vi "Decimate DFD (Array).vi"(8 "error in (no error)":errorcluster, 10 "Decimation Factor":i32, 11 "Waveforms in":waveform(dbl)[](array[waveform])) -> (0 "error out":errorcluster, 3 "waveforms out":waveform(dbl)[](array[waveform]))   [LabVIEW 2019, in "DSP.lvclass"]
uses:
  DSP.lvclass
  949379ad-8373-41eb-be01-93a6c1c1afb3.vi
  efb08f77-0c38-4651-8a9c-351b9595fc15.vi
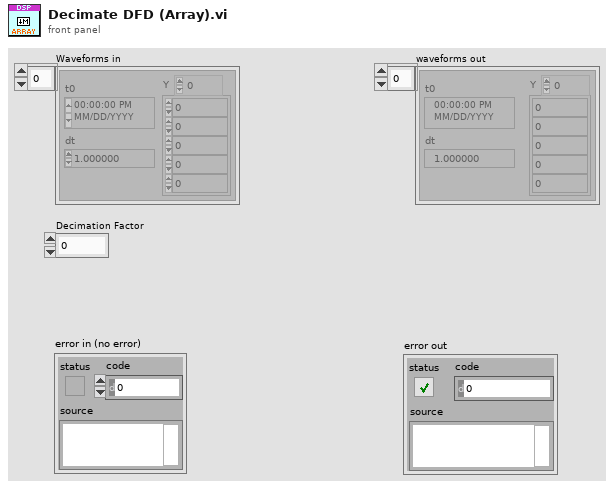
[diagram p1: front panel]
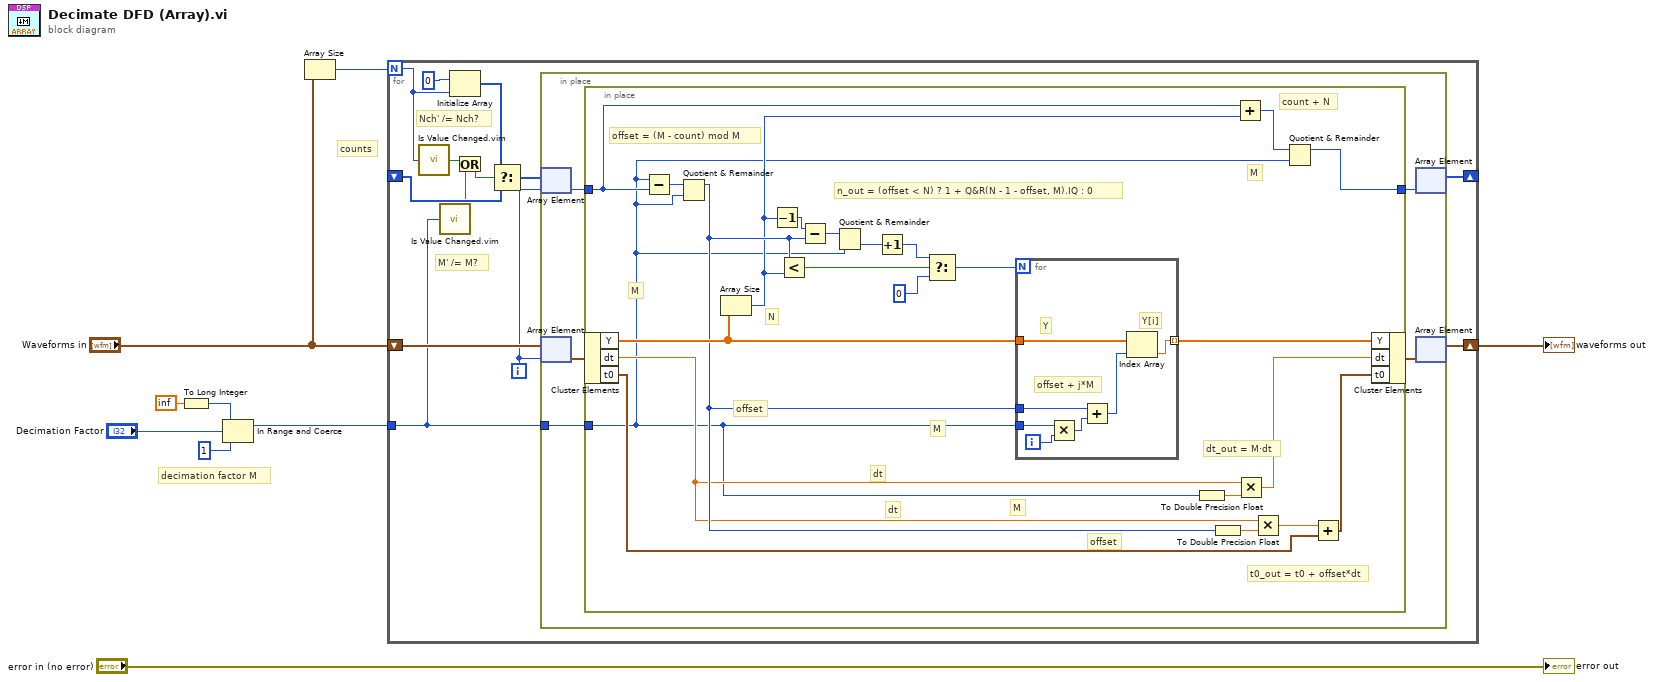
[diagram p0: block diagram]
diagram:
  # "counts"
  # "decimation factor M"
  n1 = To Long Integer(number=inf) -> (32bit integer=w4:i32)
  n2 = In Range and Coerce(upper limit=w4, x="Decimation Factor", lower limit=1) -> (coerced(x)=w2:i32)  [unwired: 1 out]
  n3 = Array Size(array="Waveforms in") -> (size(s)=w1:i32)
  n4 = for {
    N: w1 -> [w13]
    shift-right: [w21] -> w9
    shift-left: "Waveforms in" -> [w22]
    tunnel: w2 -> [w20]
    shift-right: [w16] -> _
    shift-left: _ -> [w18]
    i -> [w15]
    # "Nch' /= Nch?"
    # "M' /= M?"
    n5 = call "Is Value Changed.vim"("value"=w13) -> ("changed or first call?"=w12:bool)
    n6 = call "Is Value Changed.vim"("value"=w20) -> ("changed or first call?"=w11:bool)
    n7 = Initialize Array(0 ("disabled index (col)"), w13) -> (w19:i32[])
    n8 = Or(x=w12, y=w11) -> (x .or. y?=w10:bool)
    n9 = Select(t=w19, s=w10, f=w18) -> (s? t:f=w17:i32[])
    n10 = in-place {
      in-place-border: w20 -> [w27]
      n11 = in-place-array #1(w17, w15) -> (w24:i32)
      n12 = in-place-array #2(w22, w15) -> (w25:waveform(dbl))
      n13 = in-place {
        in-place-border: w27 -> [w28]
        in-place-border: w24 -> [w34]
        in-place-border: [w31] -> w23
        # "offset"
        # "M"
        # "dt"
        # "dt"
        # "t0_out = t0 + offset*dt"
        # "M"
        # "count + N"
        # "offset"
        # "M"
        # "n_out = (offset < N) ? 1 + Q&R(N - 1 - offset, M).IQ : 0"
        # "dt_out = M·dt"
        # "offset = (M - count) mod M"
        # "M"
        # "N"
        n14 = in-place-cluster #3(w25) -> ("Y"=w48:dbl[], "dt"=w30:dbl, "t0"=w29:timestamp)
        n15 = Subtract(x=w28, y=w34) -> (x-y=w47:i32)
        n16 = Quotient & Remainder(x=w47, y=w28) -> (x-y*floor(x/y)=w38:i32)  [unwired: 1 out]
        n17 = Array Size(array=w48) -> (size(s)=w33:i32)
        n18 = Decrement(x=w33) -> (x-1=w44:i32)
        n19 = Less?(x=w38, y=w33) -> (x < y?=w45:bool)
        n20 = Subtract(x=w44, y=w38) -> (x-y=w43:i32)
        n21 = Quotient & Remainder(x=w43, y=w28) -> (floor(x/y)=w46:i32)  [unwired: 1 out]
        n22 = Increment(x=w46) -> (x+1=w41:i32)
        n23 = Select(t=w41, s=w45, f=0) -> (s? t:f=w40:i32)
        n24 = for {
          N: w40 -> [_]
          tunnel: w48 -> [w57]
          tunnel: w28 -> [w56]
          tunnel: w38 -> [w54]
          tunnel: [w51] -> w50 mode=indexing
          i -> [w55]
          # "Y[i]"
          # "Y"
          # "offset + j*M"
          n25 = Multiply(x=w56, y=w55) -> (x*y=w53:i32)
          n26 = Add(x=w54, y=w53) -> (x+y=w52:i32)
          n27 = Index Array(array=w57, index=w52) -> (element=w51:dbl)
        }
        n28 = To Double Precision Float(number=w28) -> (double precision float=w49:dbl)
        n29 = To Double Precision Float(number=w38) -> (double precision float=w37:dbl)
        n30 = Add(x=w34, y=w33) -> (x+y=w32:i32)
        n31 = Multiply(x=w30, y=w49) -> (x*y=w39:dbl)
        n32 = Multiply(x=w30, y=w37) -> (x*y=w36:dbl)
        n33 = Quotient & Remainder(x=w32, y=w28) -> (x-y*floor(x/y)=w31:i32)  [unwired: 1 out]
        n34 = Add(x=w36, y=w29) -> (x+y=w35:timestamp)
        n35 = in-place-cluster #3("Y"=w50, "dt"=w39, "t0"=w35) -> (w26:waveform(dbl))
      }
      n36 = in-place-array #1(w23) -> (w16:i32[])  [unwired: 1 out]
      n37 = in-place-array #2(w26) -> (w21:waveform(dbl)[])  [unwired: 1 out]
    }
  }
  "waveforms out" <- w9
  "error out" <- "error in (no error)"
